vi "insert.vi"(1 "Array":i32[][](array[numeric]), 2 "AWG index":u32, 3 "cluster":T2) -> (0 "output cluster":T1)   [LabVIEW 2013]
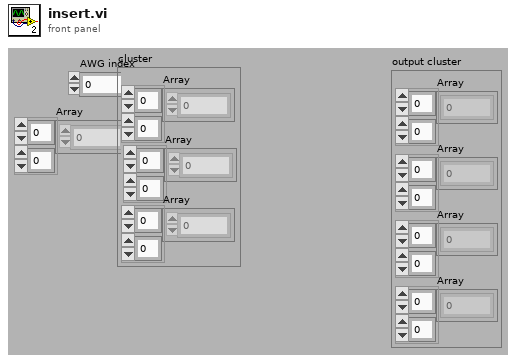
[diagram p1: front panel]
types:
  T1 = cluster{"Array":i32[][], "Array":i32[][], "Array":i32[][], "Array":i32[][]}
  T2 = cluster{"Array":i32[][], "Array":i32[][], "Array":i32[][]}
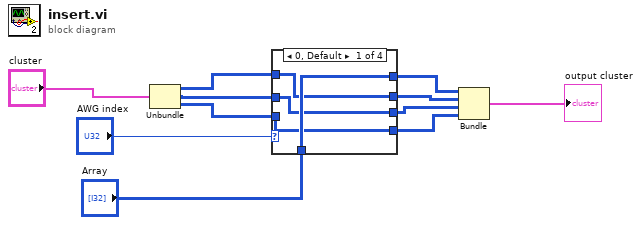
[diagram p0: block diagram]
diagram:
  n1 = Unbundle("cluster") -> ("Array"=w3:i32[][], "Array"=w2:i32[][], "Array"=w1:i32[][])
  n2 = case shown="0, Default" "AWG index" {
    tunnel: "Array" -> [w15 w19 w23 w27]
    tunnel: [w15 w18 w22 w24] -> w11
    tunnel: [w12 w19 w21 w25] -> w10
    tunnel: [w13 w16 w23 w26] -> w9
    tunnel: [w14 w17 w20 w27] -> w8
    tunnel: w3 -> [w12 w18 w22 w24]
    tunnel: w1 -> [w14 w17 w20 w26]
    tunnel: w2 -> [w13 w16 w21 w25]
    frame 0, Default {
    }
    frame 1 {
    }
    frame 2 {
    }
    frame 3 {
    }
  }
  n3 = Bundle("Array"=w11, "Array"=w10, "Array"=w9, "Array"=w8) -> (→"output cluster":T1)  [unwired: 1 in]
